vi "XW_Calib_Corr_Polysurf_PN.vi"(0 "A1 from Vel. Calib":dbl=2.21, 1 "B1 from Vel. Calib":dbl=1.36, 2 "n1 from Vel. Calib":dbl=0.42, 3 "A2 from Vel. Calib":dbl=2.25, 4 "B2 from Vel. Calib":dbl=1.4, 5 "n2 from Vel. Calib":dbl=0.41, 6 "Original XW map values":dbl[][](array[numeric]), 7 "Zero angle dataset from map (used for calib. correction)":dbl[][](array[numeric])) -> (14 "Corrected XW map values":dbl[][](array[numeric]), 18 "S*cos(q), S*sin(q), Tx, Ty":dbl[](array[numeric])=[1.0763223002323654, 0.0007524070719776288, -0.14779165640104555, -0.09827403757225917], 19 "Sx, Tx, Sy, Ty":dbl[](array[numeric])=[1.0000263372329348, -5.817138285027323e-05, 0.9999727510054321, 6.062261811624134e-05])   [LabVIEW 2011]
panel:
  # "Paul Nathan 17/02/10"
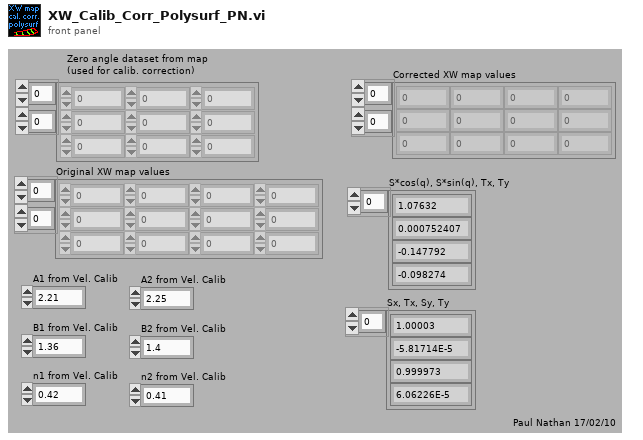
[diagram p1: front panel]
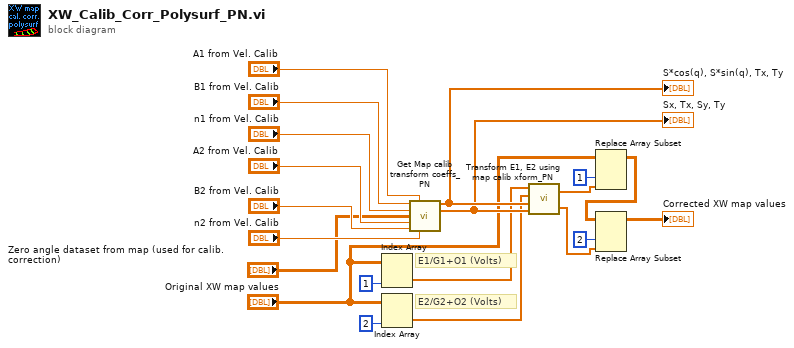
[diagram p0: block diagram]
diagram:
  # "E2/G2+O2 (Volts)"
  # "E1/G1+O1 (Volts)"
  n1 = Index Array(array="Original XW map values", index (col)=1 ("disabled index (col)")) -> (element=w10:dbl[])  [unwired: 1 in]
  n2 = Index Array(array="Original XW map values", index (col)=2 ("disabled index (col)")) -> (element=w9:dbl[])  [unwired: 1 in]
  n3 = call "Get Map calib transform coeffs_PN.vi"("B1 from Vel. Calib"="B1 from Vel. Calib", "A1 from Vel. Calib"="A1 from Vel. Calib", "n1 from Vel. Calib"="n1 from Vel. Calib", "Zero angle dataset from map (used for calib. correction)"="Zero angle dataset from map (used for calib. correction)", "A2 from Vel. Calib"="A2 from Vel. Calib", "B2 from Vel. Calib"="B2 from Vel. Calib", "n2 from Vel. Calib"="n2 from Vel. Calib") -> ("S*cos(q), S*sin(q), Tx, Ty"=w14:dbl[], "Sx, Tx, Sy, Ty"=w13:dbl[])  [unwired: 7 out]
  "S*cos(q), S*sin(q), Tx, Ty" <- w14
  "Sx, Tx, Sy, Ty" <- w13
  n4 = call "Transform E1, E2 using map calib xform_PN.vi"("Sx, Tx, Sy, Ty"=w13, "S*cos(q), S*sin(q), Tx, Ty"=w14, "E2/G2 + O2 orig"=w9, "E1/G1 + O1 orig"=w10) -> ("E2/G2 + O2 xformed"=w4:dbl[], "E1/G1 + O1 xformed"=w7:dbl[])
  n5 = Replace Array Subset(array="Original XW map values", new element=w7, index (col)=1 ("disabled index (col)")) -> (w5:dbl[][])  [unwired: 1 in]
  n6 = Replace Array Subset(array=w5, new element=w4, index (col)=2 ("disabled index (col)")) -> (→"Corrected XW map values":dbl[][])  [unwired: 1 in]
